vi "NewComponents.vi"() -> ()   [LabVIEW 2015]
panel:
  out "Removed Components":string[](array[string])
  out "Added Components":string[](array[string])
  in  "Old Component List":string[](array[string])
  in  "New Component List":string[](array[string])
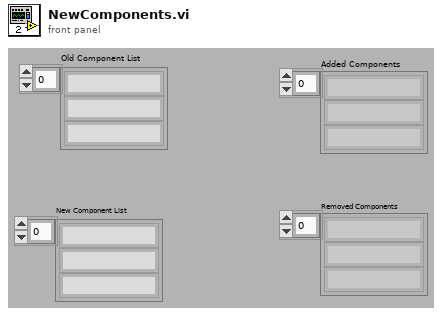
[diagram p1: front panel]
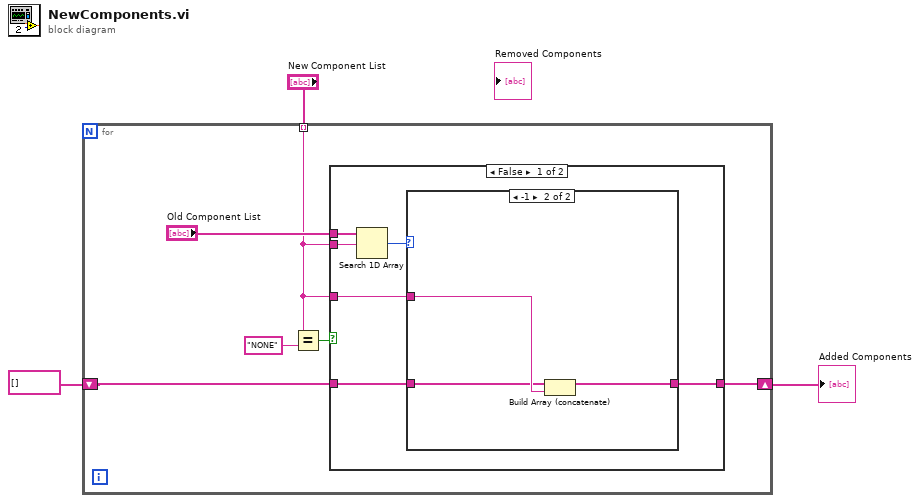
[diagram p0: block diagram]
diagram:
  n1 = for {
    shift-right: [w5] -> w1
    shift-left: string[] [] -> [w8]
    tunnel: "New Component List" -> [w4] mode=indexing
    n2 = Equal?(x=w4, y="NONE") -> (x = y?=w6:bool)
    n3 = case shown="False" w6 {
      tunnel: "Old Component List" -> [w15 _]
      tunnel: w8 -> [w13 w20]
      tunnel: w4 -> [w12 _]
      tunnel: [w10 w20] -> w5
      tunnel: w4 -> [w11 _]
      frame False {
        n4 = Search 1D Array(1D array=w15, element=w12) -> (index of element=w14:i32)  [unwired: 1 in]
        n5 = case shown="-1" w14 {
          tunnel: w13 -> [w16 w18]
          tunnel: w11 -> [_ w19]
          tunnel: [w16 w17] -> w10
          frame 0, Default {
          }
          frame -1 {
            n6 = Build Array (concatenate)(w18, w19) -> (w17:string[])
          }
        }
      }
      frame True {
      }
    }
  }
  "Added Components" <- w1
